vi "Write Mission Upload Msg.vi"(8 "error in (no error)":errorcluster, 10 "Mission":T1[](array[typedef]) {"GPS Longitude" format="%.6g"; "GPS Latitude" format="%.6g"}, 11 "Load Mission Message in":refnum<class "Mission Upload Message.lvclass">) -> (0 "error out":errorcluster, 3 "Load Mission Message out":refnum<class "Mission Upload Message.lvclass">)   [LabVIEW 2015, in "RDS Child Messages.lvlib" / "Mission Upload Message.lvclass"]
uses:
  Mission Upload Message.lvclass
  RDS Mission Controller Actor/MissionOp.ctl
  Mission Upload Message.lvclass/Mission Upload Message.ctl
  RDS Mission Controller Actor/RDS Mission Controller Actor.lvlib
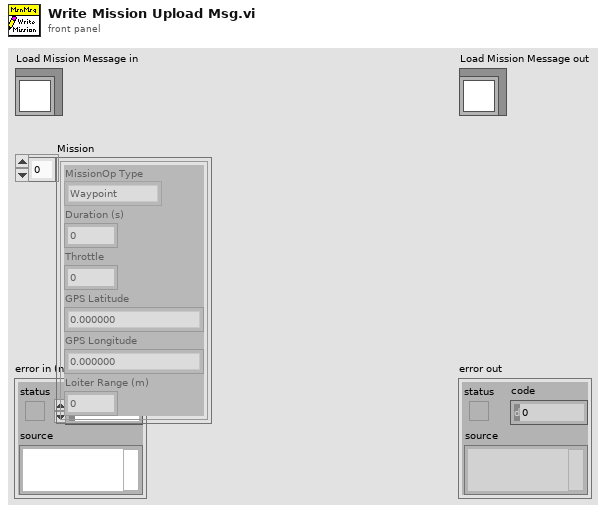
[diagram p1: front panel]
types:
  T1 = typedef "RDS Mission Controller Actor.lvlib/MissionOp.ctl" = cluster{"MissionOp Type":enum16{"Waypoint", "Loiter", "Wait", "Deploy AIP", "Stow AIP"}, "Duration (s)":u16, "Throttle":i16, "GPS Latitude":dbl, "GPS Longitude":dbl, "Loiter Range (m)":u16}
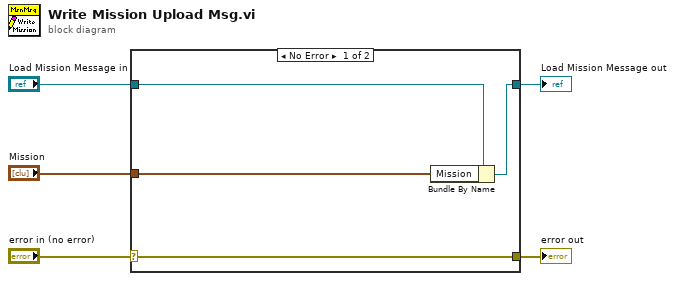
[diagram p0: block diagram]
diagram:
  n1 = case shown="No Error" "error in (no error)" {
    selector: "error in (no error)" -> [w9 w10]
    tunnel: [w9 w10] -> w4
    tunnel: [w7 w11] -> w2
    tunnel: "Load Mission Message in" -> [w8 w11]
    tunnel: "Mission" -> [w6 _]
    frame No Error {
      n2 = Bundle By Name(cluster=w8, "Mission"=w6) -> (w7:refnum<class "Mission Upload Message.lvclass">)
    }
    frame Error {
    }
  }
  "error out" <- w4
  "Load Mission Message out" <- w2
